vi "Get Weather Forecast Data.vi"(8 "error in (no error)":errorcluster, 9 "Longitude":dbl, 10 "Latitude":dbl, 11 "Weather in":refnum<class "Weather.lvclass">) -> (0 "error out":errorcluster, 3 "Weather out":refnum<class "Weather.lvclass">)   [LabVIEW 2025, in "Weather Actor.lvlib" / "Weather.lvclass"]
uses:
  Weather.lvclass
  Weather.lvclass/Weather.ctl
  UI Launcher/UI Launcher.lvlib
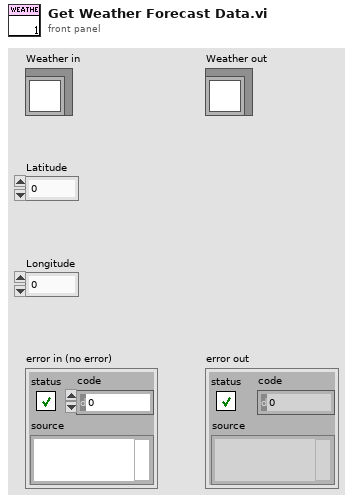
[diagram p1: front panel]
types:
  T1 = cluster{"latitude":dbl, "longitude":dbl, "generationtime_ms":dbl, "utc_offset_seconds":i32, "timezone":string, "timezone_abbreviation":string, "elevation":dbl, "current":cluster{"time":string, "interval":i32, "temperature_2m":dbl, "wind_speed_10m":dbl}, "hourly_units":cluster{"time":string, "temperature_2m":string, "wind_speed_10m":string, "relative_humidity_2m":string}, "hourly":cluster{"time":string[], "temperature_2m":dbl[], "wind_speed_10m":dbl[], "relative_humidity_2m":dbl[]}}
  T2 = cluster{timestamp[], "relative_humidity_2m":dbl[]}[]
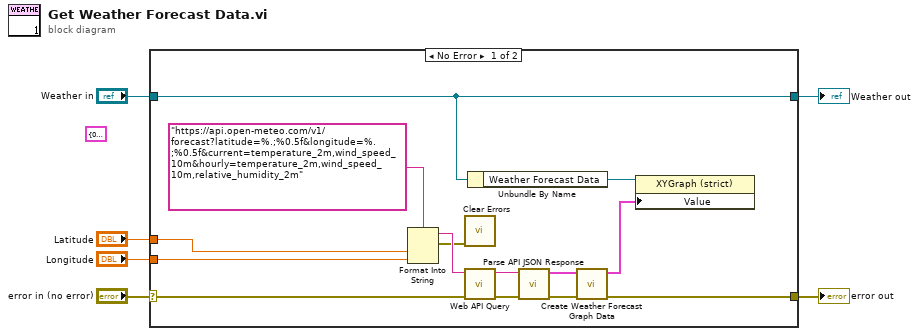
[diagram p0: block diagram]
diagram:
  (unwired) T1 {"latitude"=0.0, "longitude"=0.0, "generationtime_ms"=0.0, "utc_offset_seconds"=0, "timezone"="", "timezone_abbreviation"="", "elevation"=0.0, "current"={"time"="", "interval"=0, "temperature_2m"=0.0, "wind_speed_10m"=0.0}, "hourly_units"={"time"="", "temperature_2m"="", "wind_speed_10m"="", "relative_humidity_2m"=""}, "hourly"={"time"=[], "temperature_2m"=[], "wind_speed_10m"=[], "relative_humidity_2m"=[]}} ("Weather Forecast Data")
  n1 = case shown="No Error" "error in (no error)" {
    selector: "error in (no error)" -> [w20 w22]
    tunnel: [w11 w22] -> w5
    tunnel: [w9 w21] -> w3
    tunnel: "Weather in" -> [w9 w21]
    tunnel: "Longitude" -> [w17 _]
    tunnel: "Latitude" -> [w16 _]
    frame No Error {
      n2 = Format Into String(format string="https://api.open-meteo.com/v1/forecast?latitude=%.;%0.5f&longitude=%.;%0.5f&current=temperature_2m,wind_speed_10m&hourly=temperature_2m,wind_speed_10m,relative_humidity_2m" ("String"), w16, w17) -> (resulting string=w18:string, error out=w15:errorcluster)  [unwired: 2 in]
      n3 = call <vilib>:"Clear Errors.vi"("error in (no error)"=w15) -> ()  [unwired: 5 in, 2 out]
      n4 = call "Web API Query.vi"("error in (no error)"=w20, "url"=w18) -> ("error out"=w14:errorcluster, "API Response"=w13:string)  [unwired: 8 in]
      n5 = Unbundle By Name(w9) -> ("Weather Forecast Data"=w8:refnum<vi>)
      n6 = call "Parse API JSON Response.vi"("error in"=w14, "API Response"=w13) -> ("error out"=w12:errorcluster, "Weather Forecast Data"=w10:T1)  [unwired: 8 in]
      n7 = call "Create Weather Forecast Graph Data.vi"("error in (no error)"=w12, "Weather Forecast Response"=w10) -> ("error out"=w11:errorcluster, "Weather Forecast Data"=w7:T2)  [unwired: 8 in]
      n8 = property class="XYGraph (strict)"(reference=w8, "Value"=w7) -> ()  [unwired: 1 in, 2 out]
    }
    frame Error {
    }
  }
  "error out" <- w5
  "Weather out" <- w3
